vi "Untitled 6.vi"() -> ()   [LabVIEW 2012]
panel:
  out "Output":string
  in  "Input":string
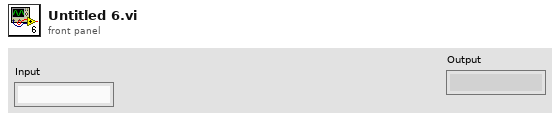
[diagram p1: front panel]
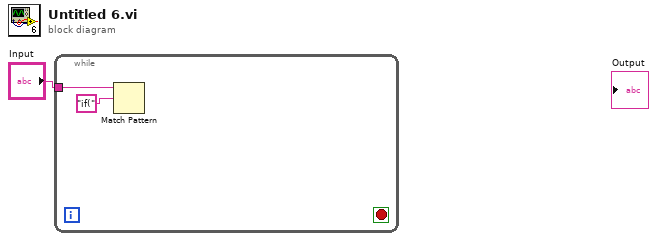
[diagram p0: block diagram]
diagram:
  n1 = while {
    tunnel: "Input" -> [w3]
    stop <- _ stop-if-true
    n2 = Match Pattern(string=w3, regular expression="if(") -> ()  [unwired: 1 in, 4 out]
  }
